vi "RPM_Calc.vi"(9 "Round":dbl, 11 "PulseSampling":string) -> (1 "Limit":dbl, 3 "delta":dbl format="%#.6f")   [LabVIEW 2017]
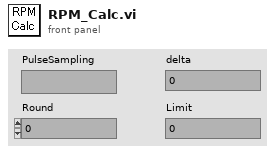
[diagram p1: front panel]
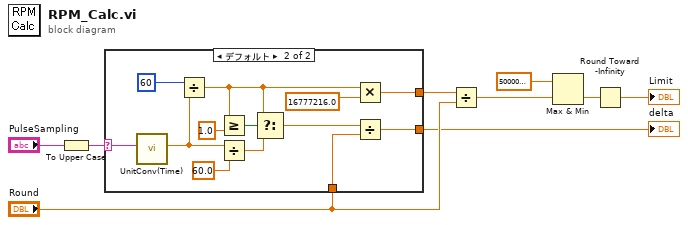
[diagram p0: block diagram]
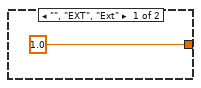
[diagram p2: hidden frame]
diagram:
  n1 = To Upper Case(1:"PulseSampling") -> (0:w8:string)
  n2 = case shown="デフォルト" w8 {
    selector: w8 -> [_ w18]
    tunnel: [1.0 w12] -> w1
    tunnel: [_ w15] -> w7
    tunnel: "Round" -> [_ w11]
    frame "", "EXT", "Ext" {
    }
    frame Default {
      n3 = call "UnitConv(Time).vi"("St IN"=w18) -> ("NumOUT"=w17:dbl)  [unwired: 3 in, 5 out]
      n4 = Divide(x=60, y=w17) -> (x/y=w16:dbl)
      n5 = Greater Or Equal?(x=w16, y=1.0) -> (x >= y?=w21:bool)
      n6 = Divide(x=w17, y=60.0) -> (x/y=w20:dbl)
      n7 = Select(t=w16, s=w21, f=w20) -> (s? t:f=w13:dbl)
      n8 = Multiply(x=w16, y=16777216.0) -> (x*y=w15:dbl)
      n9 = Divide(x=w13, y=w11) -> (x/y=w12:dbl)
    }
  }
  "delta" <- w1
  n10 = Divide(x=w7, y="Round") -> (x/y=w5:dbl)
  n11 = Max & Min(x=500000000.0 ("y"), y=w5) -> (min(x,y)=w6:dbl)  [unwired: 1 out]
  n12 = Round Toward -Infinity(1:w6) -> (0:→"Limit":dbl)
